vi "Wait For Generation Started.vi"(11 "hardware commands sync queue":T2) -> (0 "error out":errorcluster, 3 "Status":T1)   [LabVIEW 2021]
uses:
  controls/Sync Commands Queue Ref.ctl
  controls/Sync Commands.ctl
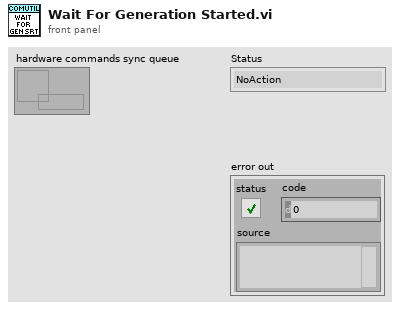
[diagram p1: front panel]
types:
  T1 = typedef "Sync Commands.ctl" = enum16{"NoAction", "GenerationStarted", "AcquisitionCompleted", "GenerationErrored"}
  T2 = typedef "Sync Commands Queue Ref.ctl" = refnum<queue>
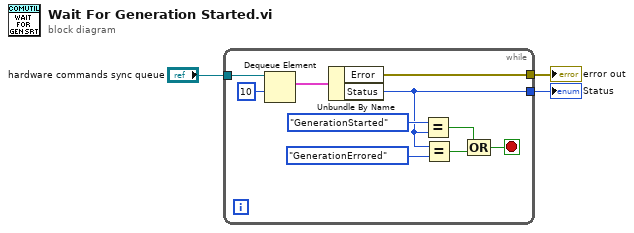
[diagram p0: block diagram]
diagram:
  n1 = while {
    tunnel: [w4] -> w1
    tunnel: "hardware commands sync queue" -> [w7]
    tunnel: [w5] -> w3
    stop <- w8 stop-if-true
    n2 = Dequeue Element(queue=w7, timeout in ms (-1)=10) -> (element=w6:cluster{"Status":T1, "Error":errorcluster})  [unwired: 1 in, 3 out]
    n3 = Unbundle By Name(w6) -> ("Error"=w5:errorcluster, "Status"=w4:T1)
    n4 = Equal?(x=Sync_Commands."GenerationStarted" ("y"), y=w4) -> (x = y?=w10:bool)
    n5 = Equal?(x=w4, y=Sync_Commands."GenerationErrored") -> (x = y?=w9:bool)
    n6 = Compound Arithmetic op=OR(w10, w9) -> (w8:bool)
  }
  "error out" <- w3
  "Status" <- w1
